vi "Traverse_Control_Ch_Names.vi"(1 "Traverse line":T1 {"Row Duration (mins)" format="%#.1f"; "Row No" min=0; "Trace Gas Concentration (%)" min=0.0 format="%#.2f"; "Emission Rate (l/min)" format="%#.2f"; "Tunnel Speed" format="%#.2f"; "Start X" format="%#.2f"; "Start Y" format="%#.2f"; "Start Z" format="%#.2f"; "End X" format="%#.2f"; "End Y" format="%#.2f"; "End Z" format="%#.2f"; "Averaging time (min)" min=0.0 format="%#.1f"}, 2 "Mode":T4(ring)) -> (0 "Channel names":string[](array[string]))   [LabVIEW 2010]
uses:
  Traverse_cluster.ctl
  Spacing.ctl
  Controls/Multi_run_mode.ctl
  Globals/Extra_Commands_Global.vi
panel:
  # "X           Y            Z"
  # "Start"
  # "End"
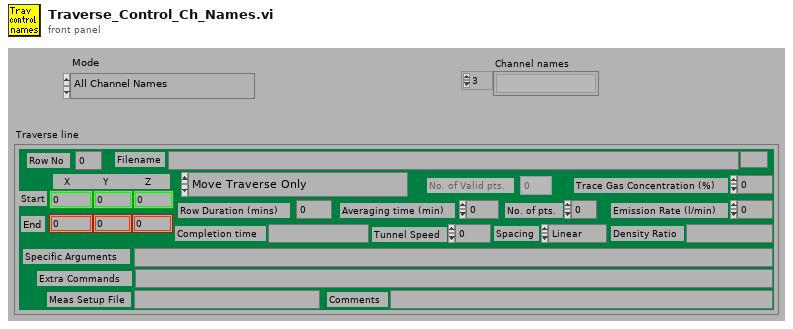
[diagram p1: front panel]
types:
  T1 = typedef "Traverse_cluster.ctl" = cluster{"Start X":dbl, "Start Y":dbl, "Start Z":dbl, "End X":dbl, "End Y":dbl, "End Z":dbl, "No. of pts.":i32, "Spacing":T2, "Filename":path, "Tunnel Speed":dbl, "Averaging time (min)":dbl, "Extra Commands":string, "Specific Arguments":string, "Emission Rate (l/min)":dbl, "Trace Gas Concentration (%)":dbl, "Density Ratio":string, "Comments":string, "Row No":i32, "Row Type Selector":T3, "Completion time":string, "Row Duration (mins)":dbl, "No. of Valid pts.":i32, "Meas Setup File":string}
  T2 = typedef "Spacing.ctl" = enum16{"Linear", "Log", "Gauss", "Specified", "N/A"}
  T3 = typedef "Multi_run_mode.ctl" = enum16{"Move Traverse Only", "Set Tunnel Speed Only", "Set Source Only", "Set Measurement Conditions", "Single Measurement", "Vertical Profile", "Lateral Profile", "Longitudinal Profile", "Explore Volume", "Multi-Axis Profile", "Auto Calibrate", "Meas Fast FID Bkgnd", "Check Beam Power", "Scanning Valve Measurement", "Run VI Named:", "Set ADAM Ch", "Wait (minutes)", "Send Message", "Synchronize With:", "Fall Back to this Row", "Turn Off Row Repeating", "Blank Row"}
  T4 = enum16{"All Channel Names", "Valid Channel Names"}
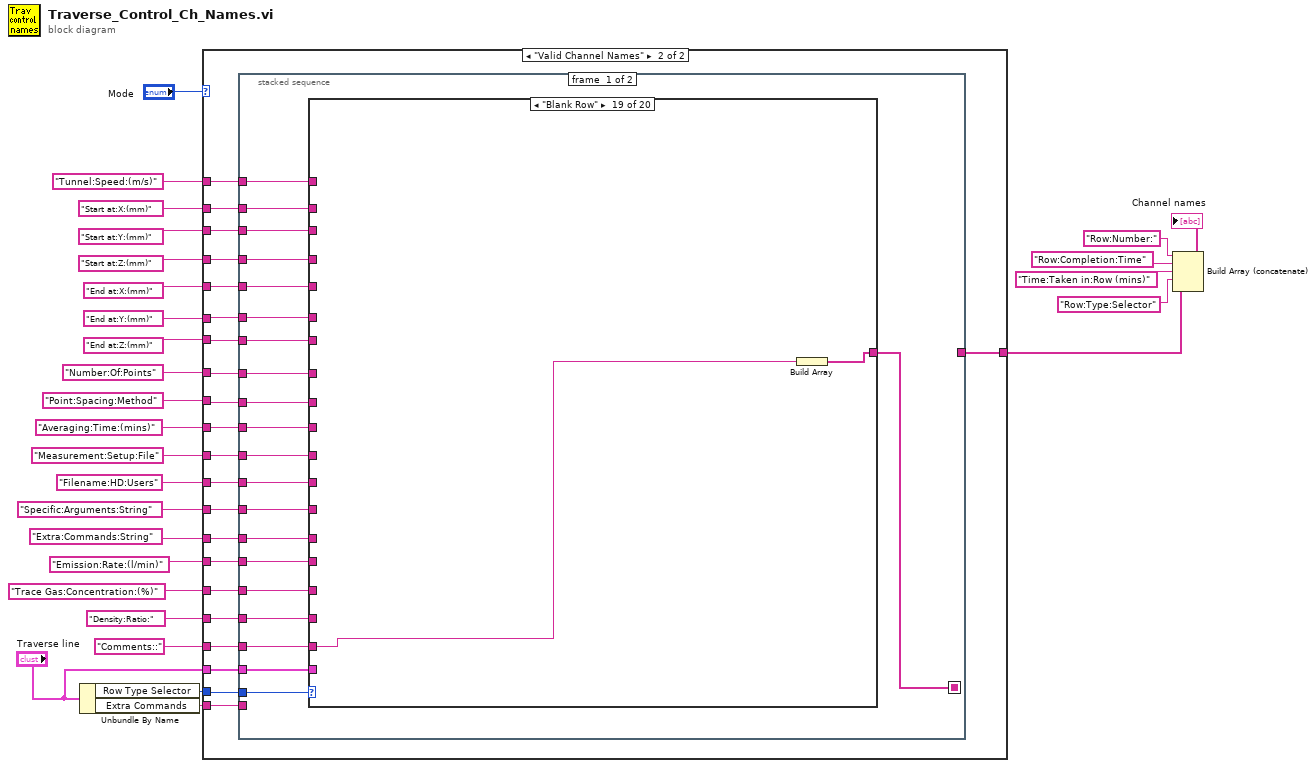
[diagram p0: block diagram]
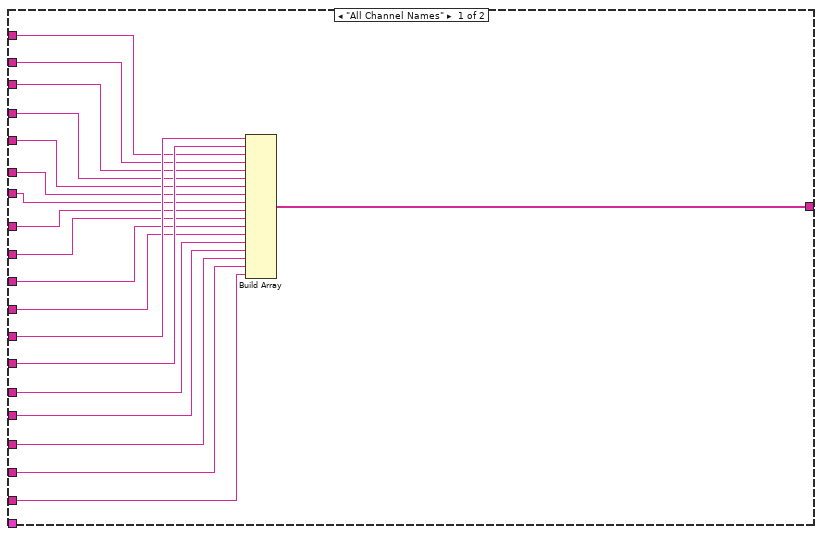
[diagram p2: hidden frame]
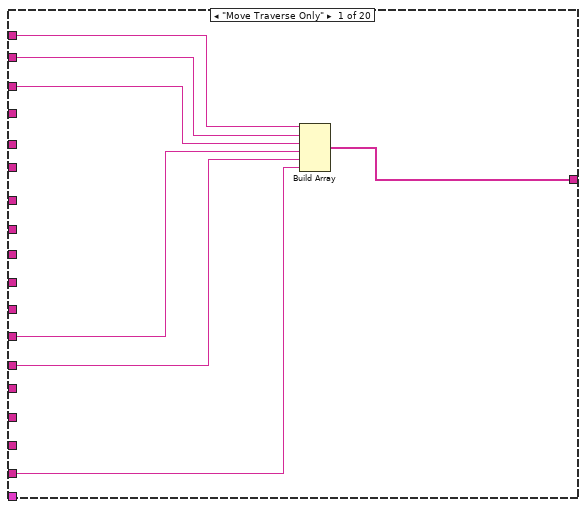
[diagram p3: hidden frame]
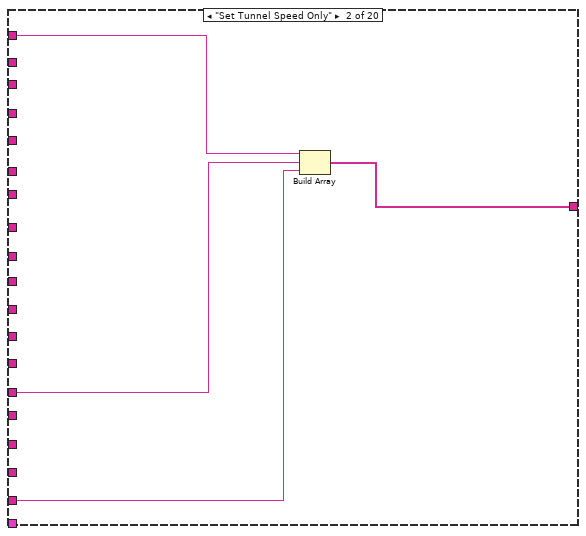
[diagram p4: hidden frame]
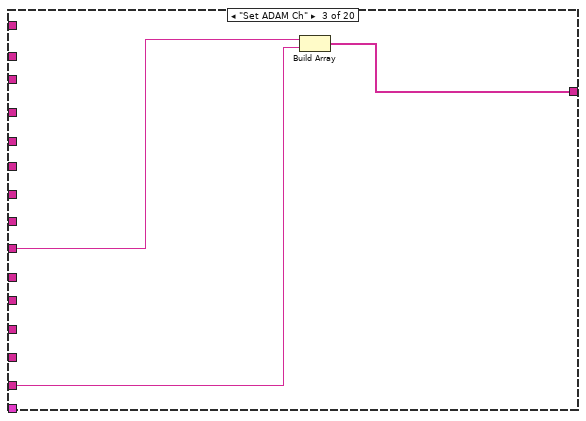
[diagram p5: hidden frame]
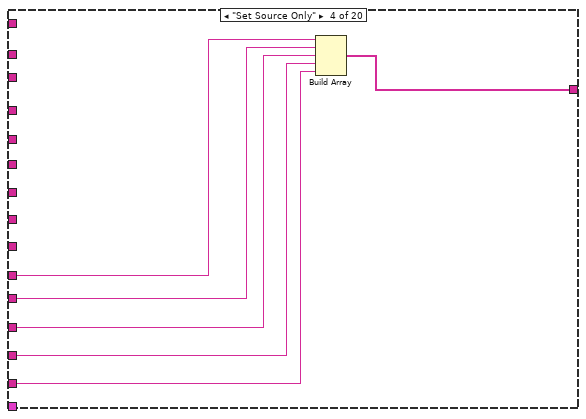
[diagram p6: hidden frame]
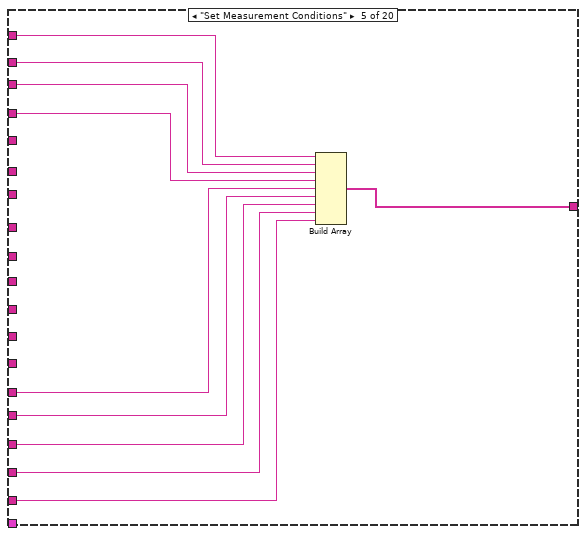
[diagram p7: hidden frame]
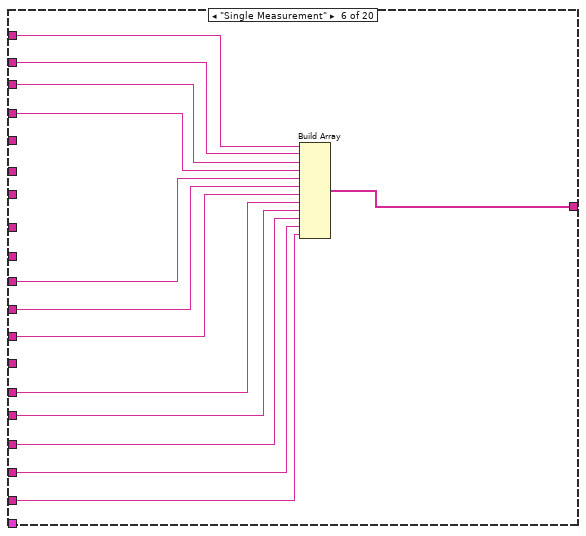
[diagram p8: hidden frame]
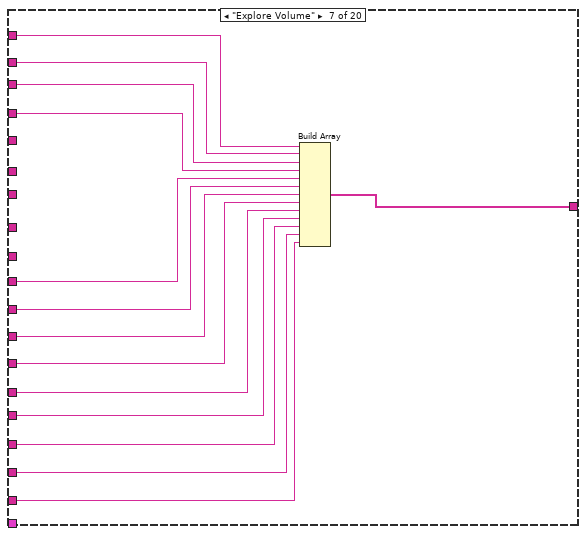
[diagram p9: hidden frame]
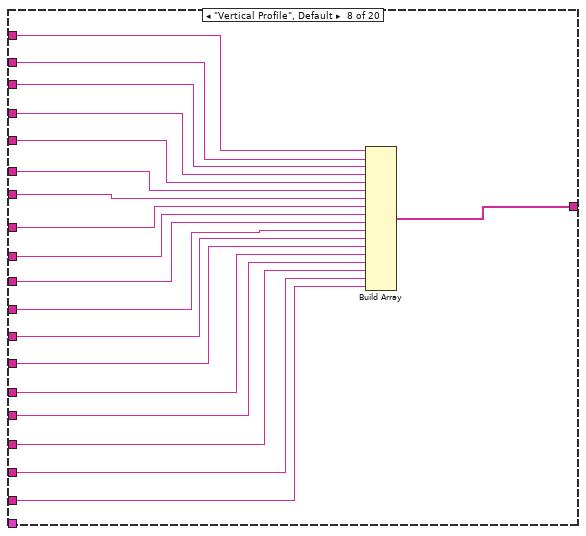
[diagram p10: hidden frame]
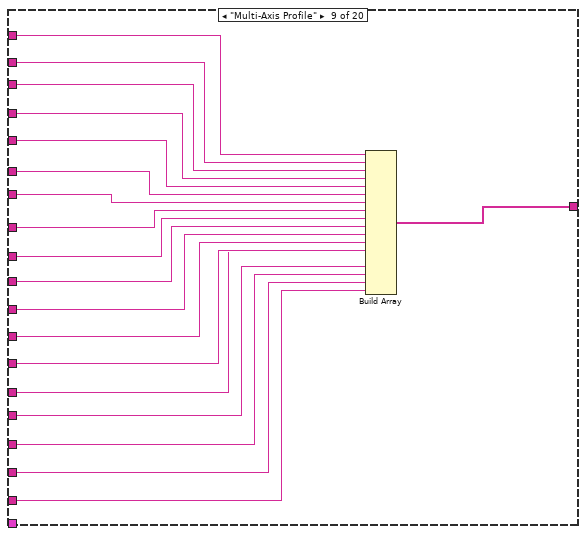
[diagram p11: hidden frame]
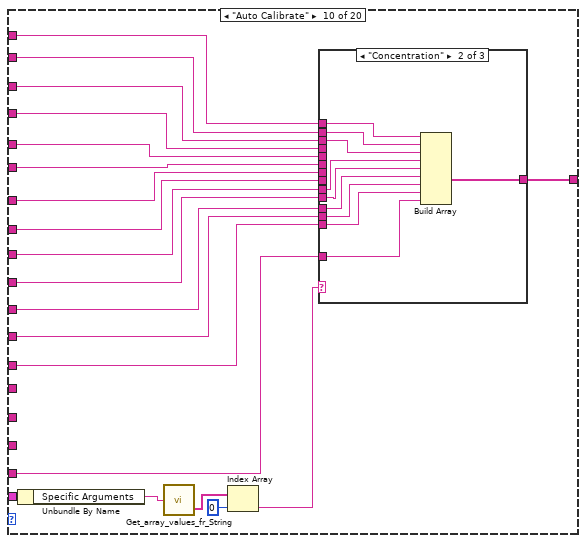
[diagram p12: hidden frame]
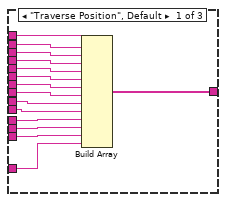
[diagram p13: hidden frame]
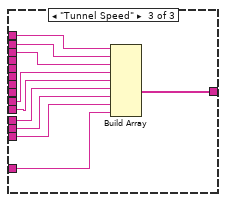
[diagram p14: hidden frame]
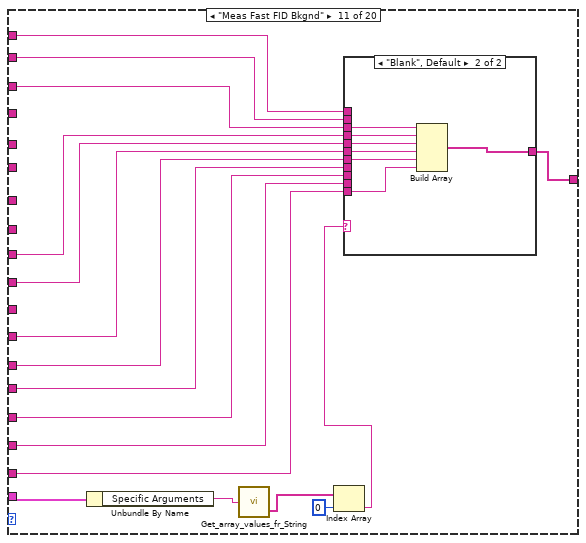
[diagram p15: hidden frame]
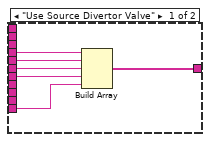
[diagram p16: hidden frame]
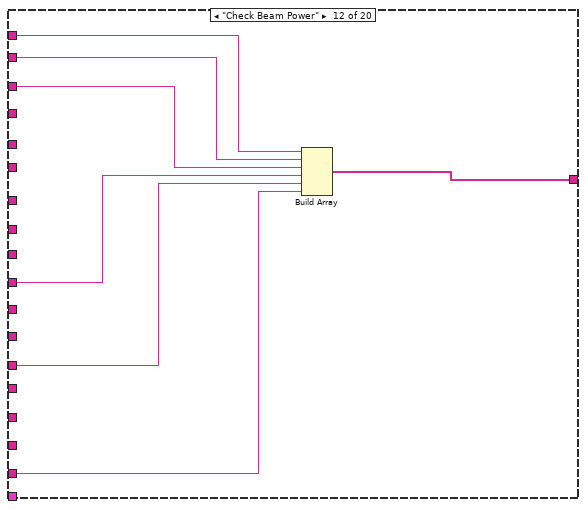
[diagram p17: hidden frame]
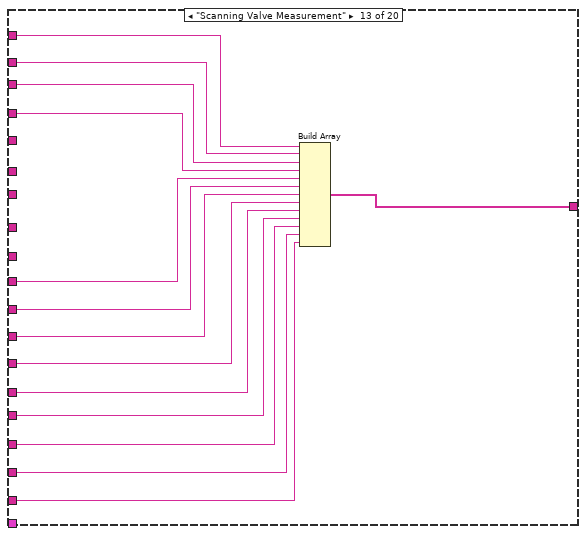
[diagram p18: hidden frame]
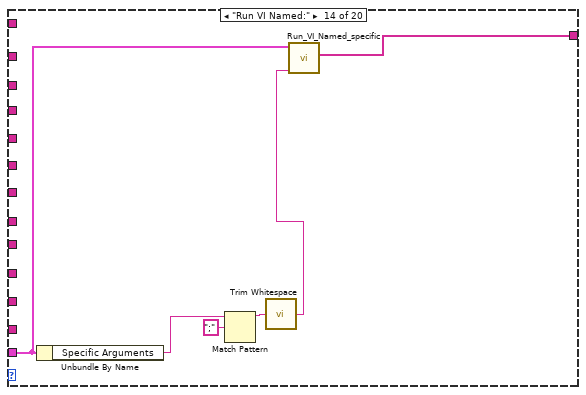
[diagram p19: hidden frame]
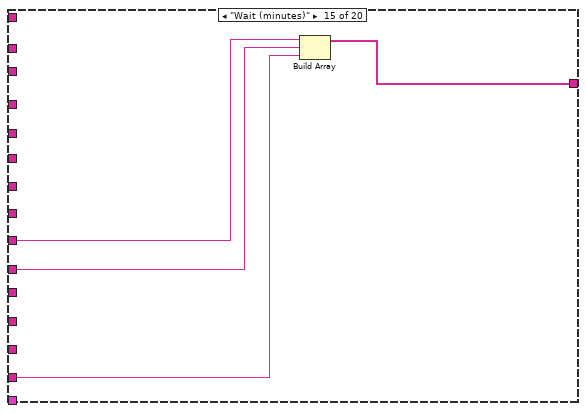
[diagram p20: hidden frame]
diagram:
  n1 = Unbundle By Name("Traverse line") -> ("Row Type Selector"=w10:T3, "Extra Commands"=w1:string)
  n2 = case shown="\"Valid Channel Names\"" "Mode" {
    tunnel: "Tunnel:Speed:(m/s)" ("Label for value") -> [w44 w68]
    tunnel: "Start at:X:(mm)" ("Label for value") -> [w43 w67]
    tunnel: "Start at:Y:(mm)" ("Label for value") -> [w42 w66]
    tunnel: "Start at:Z:(mm)" ("Label for value") -> [w41 w65]
    tunnel: "End at:X:(mm)" ("Label for value") -> [w40 w55]
    tunnel: "End at:Y:(mm)" ("Label for value") -> [w39 w54]
    tunnel: "End at:Z:(mm)" ("Label for value") -> [w38 w53]
    tunnel: "Number:Of:Points" ("Label for value") -> [w37 w52]
    tunnel: "Point:Spacing:Method" ("Label for value") -> [w36 w51]
    tunnel: "Averaging:Time:(mins)" ("Label for value") -> [w35 w57]
    tunnel: "Filename:HD:Users" ("Label for value") -> [w46 w64]
    tunnel: "Specific:Arguments:String" ("Label for value") -> [w45 w56]
    tunnel: "Extra:Commands:String" ("Label for value") -> [w34 w63]
    tunnel: "Emission:Rate:(l/min)" ("Label for value") -> [w33 w62]
    tunnel: "Trace Gas:Concentration:(%)" ("Label for value") -> [w32 w61]
    tunnel: "Density:Ratio:" ("Label for value") -> [w31 w60]
    tunnel: "Comments::" ("Label for value") -> [w30 w59]
    tunnel: w10 -> [_ w69]
    tunnel: [w47 w58] -> w6
    tunnel: "Traverse line" -> [_ w50]
    tunnel: "Measurement:Setup:File" ("Label for value") -> [w29 w49]
    tunnel: w1 -> [_ w48]
    frame "All Channel Names" {
      n3 = Build Array(w46, w45, w44, w43, w42, w41, w40, w39, w38, w37, w36, w35, w29, w34, w33, w32, w31, w30) -> (w47:string[])
    }
    frame "Valid Channel Names" {
      n4 = stacked-sequence {
        seq-local: [w70 _] -> [_ w329]
        tunnel: w69 -> [w90 _]
        tunnel: w68 -> [w89 w327]
        tunnel: w67 -> [w88 w326]
        tunnel: w66 -> [w87 w325]
        tunnel: w65 -> [w86 w324]
        tunnel: w64 -> [w85 _]
        tunnel: w63 -> [w84 _]
        tunnel: w62 -> [w83 w316]
        tunnel: w61 -> [w82 w317]
        tunnel: w60 -> [w81 w318]
        tunnel: w59 -> [w80 _]
        tunnel: [_ w330] -> w58
        tunnel: w57 -> [w79 _]
        tunnel: w56 -> [w78 _]
        tunnel: w55 -> [w77 w323]
        tunnel: w54 -> [w76 w322]
        tunnel: w53 -> [w75 w321]
        tunnel: w52 -> [w74 w320]
        tunnel: w51 -> [w73 w319]
        tunnel: w50 -> [w72 _]
        tunnel: w49 -> [w71 _]
        tunnel: w48 -> [_ w328]
        frame #0 {
          n5 = case shown="\"Blank Row\"" w90 {
            tunnel: w89 -> [_ w100 _ _ w119 w133 w147 w166 w185 _ _ _ w291 _ _ _ _ _ _ _]
            tunnel: w88 -> [w97 _ _ _ w118 w132 w146 w165 w184 w205 w253 w273 w290 _ _ _ _ _ _ _]
            tunnel: w87 -> [w96 _ _ _ w117 w131 w145 w164 w183 w204 w252 w272 w289 _ _ _ _ _ _ _]
            tunnel: w86 -> [w95 _ _ _ w116 w130 w144 w163 w182 w203 w251 w271 w288 _ _ _ _ _ _ _]
            tunnel: w85 -> [_ _ _ _ _ w127 w141 w155 w174 w196 _ _ w285 _ _ w302 _ _ _ _]
            tunnel: w84 -> [w93 w99 _ w109 w115 w122 w136 w153 w172 w194 w255 w275 w283 _ w299 w304 _ _ _ _]
            tunnel: w83 -> [_ _ _ w108 w114 w126 w140 w152 w171 _ w249 _ w282 _ _ _ _ _ _ _]
            tunnel: w82 -> [_ _ _ w107 w113 w125 w139 w151 w170 _ w248 _ w281 _ _ _ _ _ _ _]
            tunnel: w81 -> [_ _ _ w106 w112 w124 w138 w150 w169 _ w247 _ w280 _ _ _ _ _ _ _]
            tunnel: w80 -> [w92 w98 w103 w105 w111 w123 w137 w149 w168 w193 w256 w276 w279 _ w298 w303 w307 w310 w312 w315]
            tunnel: [w94 w101 w104 w110 w120 w129 w143 w162 w181 w202 w257 w277 w287 w292 w301 w306 w309 w311 w313 w314] -> w70
            tunnel: w79 -> [_ _ _ _ _ w128 w142 w156 w175 w190 w250 _ w286 _ _ _ _ _ _ _]
            tunnel: w78 -> [w91 _ w102 _ _ _ w135 w154 w173 w195 w254 _ w284 _ w300 w305 w308 _ _ _]
            tunnel: w77 -> [_ _ _ _ _ _ _ w161 w180 w201 _ _ _ _ _ _ _ _ _ _]
            tunnel: w76 -> [_ _ _ _ _ _ _ w160 w179 w200 _ _ _ _ _ _ _ _ _ _]
            tunnel: w75 -> [_ _ _ _ _ _ _ w159 w178 w199 _ _ _ _ _ _ _ _ _ _]
            tunnel: w74 -> [_ _ _ _ _ _ _ w158 w177 w198 _ _ _ _ _ _ _ _ _ _]
            tunnel: w73 -> [_ _ _ _ _ _ _ w157 w176 w197 _ _ _ _ _ _ _ _ _ _]
            tunnel: w72 -> [_ _ _ _ _ _ _ _ _ w192 w242 _ _ w293 _ _ _ _ _ _]
            tunnel: w71 -> [_ _ _ _ _ w121 w134 w148 w167 w191 w246 w274 w278 _ _ _ _ _ _ _]
            frame "Move Traverse Only" {
              n6 = Build Array(w97, w96, w95, w91, w93, w92) -> (w94:string[])
            }
            frame "Set Tunnel Speed Only" {
              n7 = Build Array(w100, w99, w98) -> (w101:string[])
            }
            frame "Set ADAM Ch" {
              n8 = Build Array(w102, w103) -> (w104:string[])
            }
            frame "Set Source Only" {
              n9 = Build Array(w109, w108, w107, w106, w105) -> (w110:string[])
            }
            frame "Set Measurement Conditions" {
              n10 = Build Array(w119, w118, w117, w116, w115, w114, w113, w112, w111) -> (w120:string[])
            }
            frame "Single Measurement" {
              n11 = Build Array(w133, w132, w131, w130, w128, w121, w127, w122, w126, w125, w124, w123) -> (w129:string[])
            }
            frame "Explore Volume" {
              n12 = Build Array(w147, w146, w145, w144, w142, w134, w141, w135, w136, w140, w139, w138, w137) -> (w143:string[])
            }
            frame "Vertical Profile", Default {
              n13 = Build Array(w166, w165, w164, w163, w161, w160, w159, w158, w157, w156, w148, w155, w154, w153, w152, w151, w150, w149) -> (w162:string[])
            }
            frame "Multi-Axis Profile" {
              n14 = Build Array(w185, w184, w183, w182, w180, w179, w178, w177, w176, w175, w167, w174, w173, w172, w171, w170, w169, w168) -> (w181:string[])
            }
            frame "Auto Calibrate" {
              n15 = Unbundle By Name(w192) -> ("Specific Arguments"=w189:string)
              n16 = call "Get_array_values_fr_String.vi"("String Value"=w189) -> ("String array"=w187:string[])  [unwired: 1 out]
              n17 = Index Array(array=w187, index=0 ("Index")) -> (element=w186:string)
              n18 = case shown="\"Concentration\"" w186 {
                tunnel: w205 -> [w220 w230 w240]
                tunnel: w204 -> [w219 w229 w239]
                tunnel: w203 -> [w218 w228 w238]
                tunnel: [w217 w227 w237] -> w202
                tunnel: w201 -> [w216 _ _]
                tunnel: w200 -> [w215 _ _]
                tunnel: w199 -> [w214 _ _]
                tunnel: w198 -> [w213 _ _]
                tunnel: w197 -> [w212 _ _]
                tunnel: w196 -> [w211 w226 w236]
                tunnel: w195 -> [w210 w225 w235]
                tunnel: w194 -> [w209 w224 w234]
                tunnel: w193 -> [w208 w223 w233]
                tunnel: w191 -> [w207 w222 w232]
                tunnel: w190 -> [w206 w221 w231]
                frame "Traverse Position", Default {
                  n19 = Build Array(w220, w219, w218, w216, w215, w214, w213, w212, w206, w207, w211, w210, w209, w208) -> (w217:string[])
                }
                frame "Concentration" {
                  n20 = Build Array(w230, w229, w228, w221, w222, w226, w225, w224, w223) -> (w227:string[])
                }
                frame "Tunnel Speed" {
                  n21 = Build Array(w240, w239, w238, w231, w232, w236, w235, w234, w233) -> (w237:string[])
                }
              }
            }
            frame "Meas Fast FID Bkgnd" {
              n22 = Unbundle By Name(w242) -> ("Specific Arguments"=w244:string)
              n23 = call "Get_array_values_fr_String.vi"("String Value"=w244) -> ("String array"=w243:string[])  [unwired: 1 out]
              n24 = Index Array(array=w243, index=0) -> (element=w241:string)
              n25 = case shown="\"Blank\", Default" w241 {
                tunnel: [w263 w270] -> w257
                tunnel: w256 -> [w262 w269]
                tunnel: w255 -> [w261 w268]
                tunnel: w254 -> [w260 w267]
                tunnel: w253 -> [_ _]
                tunnel: w252 -> [_ _]
                tunnel: w251 -> [_ w266]
                tunnel: w250 -> [w259 w265]
                tunnel: w249 -> [_ _]
                tunnel: w248 -> [_ _]
                tunnel: w247 -> [_ _]
                tunnel: w246 -> [w258 w264]
                frame "Use Source Divertor Valve" {
                  n26 = Build Array(w259, w258, w260, w261, w262) -> (w263:string[])
                }
                frame "Blank", Default {
                  n27 = Build Array(w266, w265, w264, w267, w268, w269) -> (w270:string[])
                }
              }
            }
            frame "Check Beam Power" {
              n28 = Build Array(w273, w272, w271, w274, w275, w276) -> (w277:string[])
            }
            frame "Scanning Valve Measurement" {
              n29 = Build Array(w291, w290, w289, w288, w286, w278, w285, w284, w283, w282, w281, w280, w279) -> (w287:string[])
            }
            frame "Run VI Named:" {
              n30 = Unbundle By Name(w293) -> ("Specific Arguments"=w295:string)
              n31 = Match Pattern(string=w295, regular expression=";") -> (before substring=w297:string)  [unwired: 4 out]
              n32 = call <vilib>:"Trim Whitespace.vi"("string"=w297) -> ("trimmed string"=w294:string)  [unwired: 1 in]
              n33 = call "Run_VI_Named_specific.vi"("Run VI Named String"=w294, "Multi Run Row"=w293) -> ("Channel Names"=w292:string[])  [unwired: 9 out]
            }
            frame "Wait (minutes)" {
              n34 = Build Array(w300, w299, w298) -> (w301:string[])
            }
            frame "Send Message" {
              n35 = Build Array(w302, w305, w304, w303) -> (w306:string[])
            }
            frame "Synchronize With:" {
              n36 = Build Array(w308, w307) -> (w309:string[])
            }
            frame "Fall Back to this Row" {
              n37 = Build Array(w310) -> (w311:string[])
            }
            frame "Blank Row" {
              n38 = Build Array(w312) -> (w313:string[])
            }
            frame "Turn Off Row Repeating" {
              n39 = Build Array(w315) -> (w314:string[])
            }
          }
        }
        frame #1 {
          n40 = Empty String/Path?(string/path=w328) -> (empty?=w331:bool)
          n41 = case shown="True" w331 {
            tunnel: [w332 w390] -> w330
            tunnel: w329 -> [w334 w390]
            tunnel: w328 -> [w338 _]
            tunnel: w327 -> [w345 _]
            tunnel: w326 -> [w357 _]
            tunnel: w325 -> [w356 _]
            tunnel: w324 -> [w355 _]
            tunnel: w323 -> [w354 _]
            tunnel: w322 -> [w353 _]
            tunnel: w321 -> [w352 _]
            tunnel: w320 -> [w351 _]
            tunnel: w319 -> [w350 _]
            tunnel: w318 -> [w343 _]
            tunnel: w317 -> [w342 _]
            tunnel: w316 -> [w341 _]
            frame False {
              n42 = global read "Extra_Commands_Global.vi" "Skip Traverse Position Demand"() -> (w358:string)
              n43 = global read "Extra_Commands_Global.vi" "Skip Tunnel Speed Demand"() -> (w347:string)
              n44 = Match Pattern(string=w338, regular expression=w358) -> (offset past match=w359:i32)  [unwired: 4 out]
              n45 = global read "Extra_Commands_Global.vi" "Skip Source Demand"() -> (w337:string)
              n46 = Match Pattern(string=w338, regular expression=w347) -> (offset past match=w348:i32)  [unwired: 4 out]
              n47 = Greater Than 0?(x=w359) -> (x > 0?=w349:bool)
              n48 = case shown="True" w349 {
                tunnel: w357 -> [_ w389]
                tunnel: w356 -> [_ w388]
                tunnel: w355 -> [_ w387]
                tunnel: w354 -> [_ w386]
                tunnel: w353 -> [_ w385]
                tunnel: w352 -> [_ w384]
                tunnel: w351 -> [_ w383]
                tunnel: w350 -> [_ w382]
                tunnel: [string[] [] w381] -> w344
                frame False {
                }
                frame True {
                  n49 = Build Array(w389, w388, w387, w386, w385, w384, w383, w382) -> (w381:string[])
                }
              }
              n50 = Greater Than 0?(x=w348) -> (x > 0?=w346:bool)
              n51 = case shown="True" w346 {
                tunnel: w345 -> [_ w379]
                tunnel: w344 -> [w376 w378]
                tunnel: [w376 w377] -> w340
                frame False {
                }
                frame True {
                  n52 = Build Array (concatenate)(w379, w378) -> (w377:string[])
                }
              }
              n53 = Match Pattern(string=w338, regular expression=w337) -> (offset past match=w339:i32)  [unwired: 4 out]
              n54 = Greater Than 0?(x=w339) -> (x > 0?=w336:bool)
              n55 = case shown="False" w336 {
                tunnel: w341 -> [_ w375]
                tunnel: w342 -> [_ w374]
                tunnel: w343 -> [_ w373]
                tunnel: [w370 w372] -> w335
                tunnel: w340 -> [w370 w371]
                frame False {
                }
                frame True {
                  n56 = Build Array (concatenate)(w371, w375, w374, w373) -> (w372:string[])
                }
              }
              n57 = for {
                shift-right: [w360] -> w332
                shift-left: string[] [] -> [w362]
                tunnel: w335 -> [w365]
                tunnel: w334 -> [w361] mode=indexing
                n58 = Search 1D Array(1D array=w365, element=w361) -> (index of element=w364:i32)  [unwired: 1 out]
                n59 = Less Than 0?(x=w364) -> (x < 0?=w363:bool)
                n60 = case shown="True" w363 {
                  tunnel: w362 -> [w366 w369]
                  tunnel: w361 -> [_ w368]
                  tunnel: [w366 w367] -> w360
                  frame False {
                  }
                  frame True {
                    n61 = Build Array (concatenate)(w369, w368) -> (w367:string[])
                  }
                }
              }
            }
            frame True {
            }
          }
        }
      }
    }
  }
  n62 = Build Array (concatenate)("Row:Number:" ("Label for value"), "Row:Completion:Time" ("Label for value"), "Time:Taken in:Row (mins)" ("Label for value"), "Row:Type:Selector" ("Label for value"), w6) -> (→"Channel names":string[])
